vi "read.vi"(8 "error in (no error)":errorcluster, 10 "ElectrometerController in":refnum<class "ElectrometerController.lvclass">, 11 "State in":refnum<class "ElectrometerState.lvclass">) -> (0 "error out":errorcluster, 1 "lastMeasure":dbl, 2 "ElectrometerController out":refnum<class "ElectrometerController.lvclass">, 3 "State out":refnum<class "ElectrometerState.lvclass">, 4 "newValue":bool)   [LabVIEW 2016, in "ElectrometerState.lvclass"]
uses:
  ElectrometerState.lvclass
  ElectrometerController/ElectrometerController.lvclass
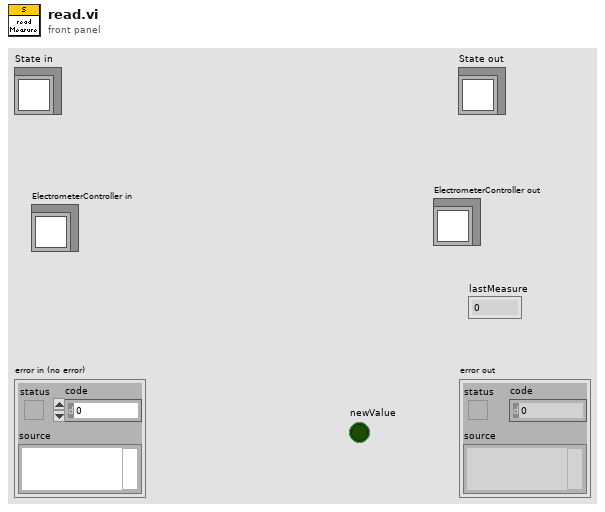
[diagram p1: front panel]
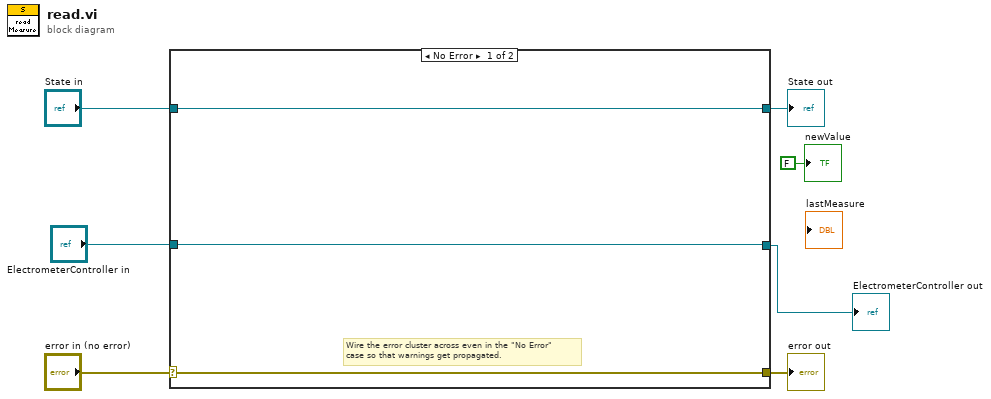
[diagram p0: block diagram]
diagram:
  n1 = case shown="No Error" "error in (no error)" {
    selector: "error in (no error)" -> [w9 w13]
    tunnel: [w9 w13] -> w6
    tunnel: [w10 w12] -> w4
    tunnel: "State in" -> [w10 w12]
    tunnel: [w8 w11] -> w2
    tunnel: "ElectrometerController in" -> [w8 w11]
    frame No Error {
      # "Wire the error cluster across even in the \"No Error\"\ncase so that warnings get propagated."
    }
    frame Error {
    }
  }
  "error out" <- w6
  "State out" <- w4
  "ElectrometerController out" <- w2
  "newValue" <- FALSE ("newValue")
